vi "Asylum_WriteGroup.vi"(8 "error in (no error)":errorcluster, 9 "groupName":string, 10 "wave":string, 11 "Application":refnum<k7>) -> (0 "error out":errorcluster, 3 "Application":refnum<k7>)   [LabVIEW 2020]
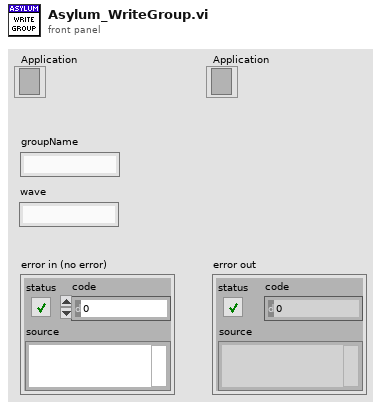
[diagram p1: front panel]
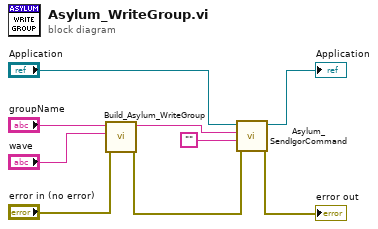
[diagram p0: block diagram]
diagram:
  n1 = call "Build_Asylum_WriteGroup.vi"("error in (no error)"="error in (no error)", "wave"="wave", "groupName"="groupName") -> ("error out"=w9:errorcluster, "Command"=w7:string)  [unwired: 7 in]
  n2 = call "Asylum_SendIgorCommand.vi"("error in (no error)"=w9, "Format"="", "command"=w7, "Application"="Application") -> ("error out"=→"error out":errorcluster, "Application"=→"Application":refnum<k7>)  [unwired: 4 in, 2 out]
